vi "Add-UpdateSailingPoints.vi"(7 "Has the first mission changed?":bool, 9 "NotifierReff":T1, 10 "Mission Notifiers":T2, 11 "Waypoints queue for Midbrain":refnum<queue>) -> (1 "Number of sailing points added":i32, 2 "Added sailing points?":bool, 3 "Added intermediate point?":bool)   [LabVIEW 2013]
uses:
  Classes/Waypoint/Waypoint.lvclass
  Data/TypeDefs/MissionNotifiers.ctl
  Classes/Missions/GenericMission/GenericMission.lvclass
  Classes/Obstacle/Obstacle.lvclass
  Data/TypeDefs/Notifiers.ctl
  Data/TypeDefs/UTM Location.ctl
  Data/TypeDefs/Sail Set Suggestions.ctl
  Data/TypeDefs/Rudder Set Suggestions.ctl
  Data/TypeDefs/OverrideInformation.ctl
  Data/TypeDefs/OverrideMode.ctl
  Data/TypeDefs/MotorSetup.ctl
  Data/TypeDefs/DynamixelSetupInfo.ctl
  Data/TypeDefs/AirmarStatus.ctl
  Data/TypeDefs/HardwareOnline.ctl
  Data/TypeDefs/DynamixelCycleTracker.ctl
  Data/TypeDefs/RC Input Values.ctl
  Utilities/Math/Angles/Angle/Angle.lvclass
panel:
  in  "Cutoff wind shift for recalc (deg) (10)":dbl=10.0
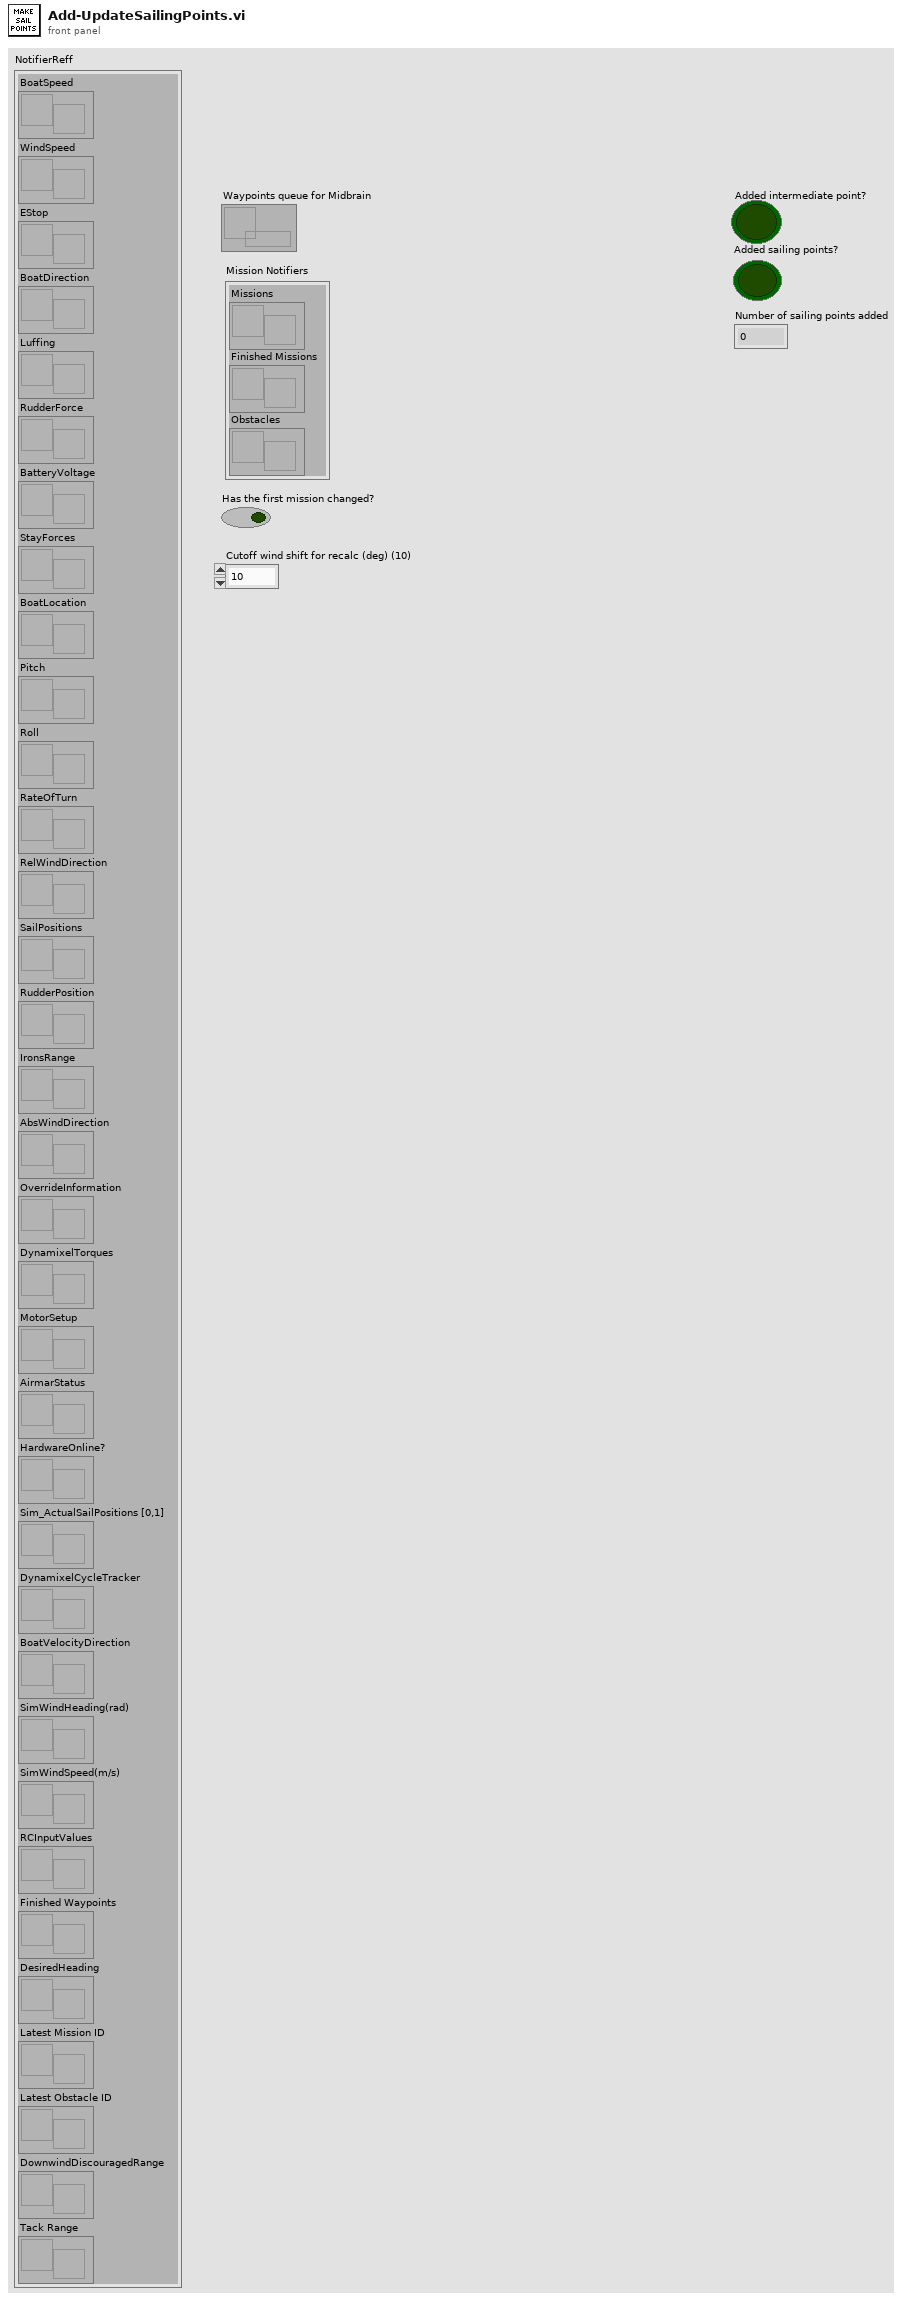
[diagram p1: front panel]
types:
  T1 = typedef "Notifiers.ctl" = cluster{"BoatSpeed":refnum<notifier>, "WindSpeed":refnum<notifier>, "EStop":refnum<notifier>, "BoatDirection":refnum<notifier>, "Luffing":refnum<notifier>, "RudderForce":refnum<notifier>, "BatteryVoltage":refnum<notifier>, "StayForces":refnum<notifier>, "BoatLocation":refnum<notifier>, "Pitch":refnum<notifier>, "Roll":refnum<notifier>, "RateOfTurn":refnum<notifier>, "RelWindDirection":refnum<notifier>, "SailPositions":refnum<notifier>, "RudderPosition":refnum<notifier>, "IronsRange":refnum<notifier>, "AbsWindDirection":refnum<notifier>, "OverrideInformation":refnum<notifier>, "DynamixelTorques":refnum<notifier>, "MotorSetup":refnum<notifier>, "AirmarStatus":refnum<notifier>, "HardwareOnline?":refnum<notifier>, "Sim_ActualSailPositions [0,1]":refnum<notifier>, "DynamixelCycleTracker":refnum<notifier>, "BoatVelocityDirection":refnum<notifier>, "SimWindHeading(rad)":refnum<notifier>, "SimWindSpeed(m/s)":refnum<notifier>, "RCInputValues":refnum<notifier>, "Finished Waypoints":refnum<notifier>, "DesiredHeading":refnum<notifier>, "Latest Mission ID":refnum<notifier>, "Latest Obstacle ID":refnum<notifier>, "DownwindDiscouragedRange":refnum<notifier>, "Tack Range":refnum<notifier>}
  T2 = typedef "MissionNotifiers.ctl" = cluster{"Missions":refnum<notifier>, "Finished Missions":refnum<notifier>, "Obstacles":refnum<notifier>}
  T3 = typedef "UTM Location.ctl" = cluster{"UTM Zone":dbl, "Hemisphere":enum16{"North", "South"}, "East":dbl, "North":dbl}
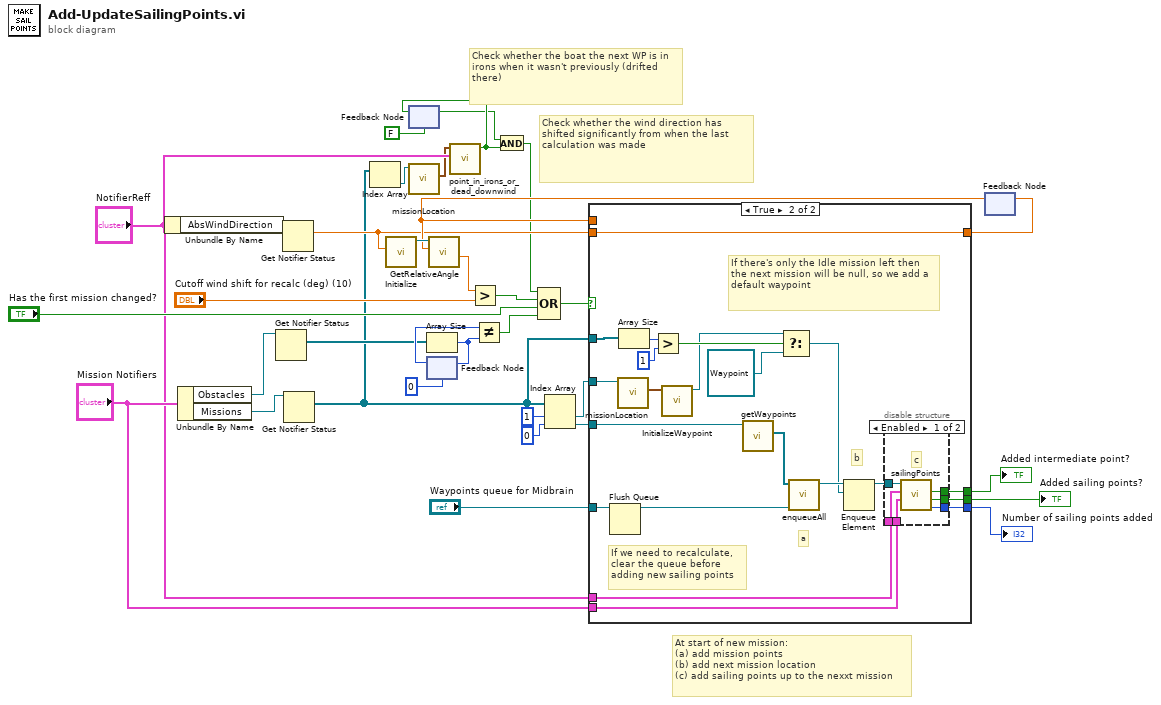
[diagram p0: block diagram]
diagram:
  # "Check whether the wind direction has shifted significantly from when the last calculation was made"
  # "Check whether the boat the next WP is in irons when it wasn't previously (drifted there)"
  # "At start of new mission:\n(a) add mission points\n(b) add next mission location\n(c) add sailing points up to the nexxt mission"
  n1 = Unbundle By Name("NotifierReff") -> ("AbsWindDirection"=w29:refnum<notifier>)
  n2 = Unbundle By Name("Mission Notifiers") -> ("Obstacles"=w7:refnum<notifier>, "Missions"=w8:refnum<notifier>)
  n3 = Get Notifier Status(notifier=w7) -> (current notification=w11:refnum<class "Obstacle.lvclass">[])  [unwired: 1 in, 4 out]
  n4 = Get Notifier Status(notifier=w29) -> (current notification=w20:dbl)  [unwired: 1 in, 4 out]
  n5 = Get Notifier Status(notifier=w8) -> (current notification=w1:refnum<class "GenericMission.lvclass">[])  [unwired: 1 in, 4 out]
  n6 = Index Array(array=w1) -> (element=w10:refnum<class "GenericMission.lvclass">)  [unwired: 1 in]
  n7 = call "Initialize.vi"("Input Angle (Deg.)"=w20) -> ("Angle out"=w23:refnum<class "Angle.lvclass">)  [unwired: 9 in, 1 out]
  n8 = feedback #1(FALSE ("In irons or dead downwind?")) -> (w13:bool)
  n9 = call-dynamic "missionLocation.vi"("GenericMission in"=w10) -> ("element"=w9:T3)  [unwired: 8 in, 2 out]
  n10 = Array Size(array=w11) -> (size(s)=w27:i32)
  n11 = feedback-in #2(w27) -> ()
  n12 = feedback #2(0) -> (w28:i32)
  n13 = call "point_in_irons_or_dead_downwind.vi"("NotifierReff"="NotifierReff", "Point"=w9) -> ("In irons or dead downwind?"=w14:bool)  [unwired: 7 in, 2 out]
  n14 = feedback-in #1(w14) -> ()
  n15 = Not Equal?(x=w28, y=w27) -> (x != y?=w26:bool)
  n16 = And(x=w13, y=w14) -> (x .and. y?=w12:bool)
  n17 = Index Array(array=w1, index #1=1 ("index"), index #2=0 ("index")) -> (element #1=w32:refnum<class "GenericMission.lvclass">, element #2=w33:refnum<class "GenericMission.lvclass">)
  n18 = feedback #3() -> (w21:dbl)  [unwired: 1 in]
  n19 = call "GetRelativeAngle.vi"("Boat Heading (Deg.)"=w21, "Angle in"=w23) -> ("Absolute difference (deg)"=w18:dbl)  [unwired: 6 in, 3 out]
  n20 = Greater?(x=w18, y="Cutoff wind shift for recalc (deg) (10)") -> (0:w17:bool)
  n21 = Compound Arithmetic op=OR(w12, w17, "Has the first mission changed?", w26) -> (w24:bool)
  n22 = case shown="True" w24 {
    tunnel: w33 -> [_ w56]
    tunnel: w32 -> [_ w54]
    tunnel: "Waypoints queue for Midbrain" -> [_ w50]
    tunnel: [w35 w51] -> w22
    tunnel: w21 -> [w35 _]
    tunnel: w20 -> [_ w51]
    tunnel: "NotifierReff" -> [_ w48]
    tunnel: "Mission Notifiers" -> [_ w47]
    tunnel: [_ w46] -> w6
    tunnel: [_ w45] -> w5
    tunnel: [_ w44] -> w4
    tunnel: w1 -> [_ w39]
    frame False {
    }
    frame True {
      # "If there's only the Idle mission left then the next mission will be null, so we add a default waypoint"
      # "If we need to recalculate, clear the queue before adding new sailing points"
      # "a"
      # "b"
      n23 = Flush Queue(queue=w50) -> (queue out=w49:refnum<queue>)  [unwired: 1 in, 2 out]
      n24 = call-dynamic "missionLocation.vi"("GenericMission in"=w54) -> ("element"=w52:T3)  [unwired: 8 in, 2 out]
      n25 = Array Size(array=w39) -> (size(s)=w42:i32)
      n26 = Greater?(x=w42, y=1) -> (0:w41:bool)
      n27 = call "InitializeWaypoint.vi"("Coords"=w52) -> ("Waypoint Out"=w38:refnum<class "Waypoint.lvclass">)  [unwired: 10 in]
      n28 = call-dynamic "getWaypoints.vi"("GenericMission in"=w56) -> ("Waypoint Array"=w55:refnum<class "Waypoint.lvclass">[])  [unwired: 8 in, 2 out]
      n29 = Select(t=w38, s=w41, f=refnum<class "Waypoint.lvclass"> refnum) -> (s? t:f=w36:refnum<class "Waypoint.lvclass">)
      n30 = call "enqueueAll.vi"("Waypoint Queue"=w49, "Waypoint Array"=w55) -> ("Waypoint Queue Out"=w53:refnum<queue>)  [unwired: 9 in]
      n31 = Enqueue Element(queue=w53, element=w36) -> (queue out=w43:refnum<queue>)  [unwired: 2 in, 2 out]
      n32 = disable-structure shown="Enabled" {
        disable-tunnel: w48 -> [w62 _]
        disable-tunnel: w47 -> [w61 _]
        disable-tunnel: [w60 _] -> w46
        disable-tunnel: [w59 _] -> w45
        disable-tunnel: [w58 _] -> w44
        disable-tunnel: w43 -> [w57 _]
        frame Enabled {
          # "c"
          n33 = call "sailingPoints.vi"("Mission Notifiers"=w61, "NotifierReff"=w62, "Waypoint queue"=w57) -> ("Number of sailing points added"=w58:i32, "Added sailing points?"=w59:bool, "Added intermediate point?"=w60:bool)  [unwired: 5 in, 1 out]
        }
        frame Disabled {
        }
      }
    }
  }
  "Added intermediate point?" <- w6
  "Added sailing points?" <- w5
  "Number of sailing points added" <- w4
  n34 = feedback-in #3(w22) -> ()
